vi "Get All.vi"(8 "error in (no error)":errorcluster, 11 "Dictionary in":refnum<class "Dictionary.lvclass">) -> (0 "error out":errorcluster, 1 "Keys":variant[](array[variant]), 2 "Names":string[](array[string]), 3 "Dictionary out":refnum<class "Dictionary.lvclass">)   [LabVIEW 2018, in "Application.lvlib" / "Dictionary.lvclass"]
uses:
  Dictionary.lvclass
  Dictionary.lvclass/Dictionary.ctl
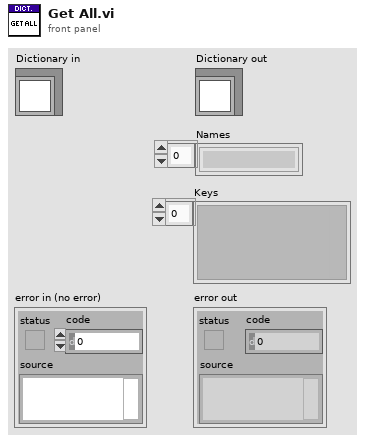
[diagram p1: front panel]
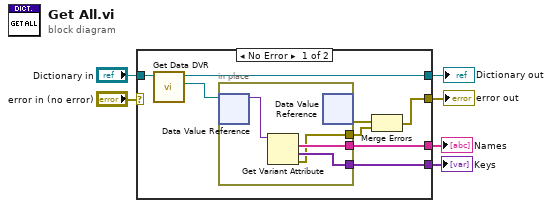
[diagram p0: block diagram]
diagram:
  n1 = case shown="No Error" "error in (no error)" {
    selector: "error in (no error)" -> [_ w20]
    tunnel: [w7 w20] -> w5
    tunnel: [w12 w19] -> w3
    tunnel: "Dictionary in" -> [w14 w19]
    tunnel: [w11 _] -> w2
    tunnel: [w10 _] -> w1
    frame No Error {
      n2 = call "Get Data DVR.vi"("Dictionary in"=w14) -> ("Data DVR"=w13:refnum<data-value>, "Dictionary out"=w12:refnum<class "Dictionary.lvclass">)  [unwired: 8 in, 1 out]
      n3 = in-place {
        in-place-border: [w17] -> w11
        in-place-border: [w16] -> w10
        in-place-border: [w15] -> w8
        n4 = in-place-dvr #1(w13) -> (w18:variant)  [unwired: 1 out]
        n5 = Get Variant Attribute(Variant=w18) -> (names=w17:string[], values=w16:variant[], error out=w15:errorcluster)  [unwired: 3 in, 1 out]
        n6 = in-place-dvr #1() -> (w9:errorcluster)  [unwired: 1 in, 1 out]
      }
      n7 = Merge Errors(w9, w8) -> (w7:errorcluster)
    }
    frame Error {
    }
  }
  "error out" <- w5
  "Dictionary out" <- w3
  "Names" <- w2
  "Keys" <- w1
